vi "fgv_Sys Config.vi"(7 "Standalone viewer initialisation?":bool, 8 "error in (no error)":errorcluster, 10 "Function":T11, 11 "System Config in":T1={"XY Stage"={"COM port"="", "XY stage available"=FALSE, "Baudrate"=0, "Type"=""}, "DAQ FPGA"={"Target"="RIO0", "input card type"=enum."AC Card", "Ref"=refnum, "Clock Freq (MHz) "=200.0, "Samples Wait after Trigger"=5080, "AOD fill"=4900, "StartupDelay"=0, "Slip Cycle (clock cycles)"=600000, "Add Cycle"=TRUE}, "Control system"={"Ctrl FPGA available"=FALSE, "Control system.FPGA Type"="", "Control system.Network adapter name"="", "Control system.MAC address"="", "Control system.Ethernet Port"=3, "Ethernet opened"=FALSE, "Ctrl FPGA Clock (MHz)"=240.0, "AOD 1 Amplitude"=0, "AOD 2 Amplitude"=0, "AOD 3 Amplitude"=0, "AOD 4 Amplitude"=0, "AOD 5 Amplitude"=0, "AOD 6 Amplitude"=0, "Data Time Interval (ns)"=0.0, "T0 (ns)"=0.0, "Ta (ns)"=0.0, "Ethernet Port"=3}, "Encoder"={"IP address"="224.0.1.103", "Port"=7000, "Encoder available"=FALSE, "Wheel radius (cm)"=16.0, "Encoder Trigger"=""}, "DAQmx Chan"={"Pockels AO"="", "Hard shutter AO"="", "PMT AOs"="", "Galvo AOs"="", "Power meter AI"=""}, "Computer MAC address"="", "Cam VidRec"={"DO flag-Video record"="", "DO flag-Trial start"="", "VidRec available"=FALSE}, "Externalise Triggers"=FALSE, "MC Supported"=FALSE, "Laser wavelength (nm)"=920.0} {"Laser wavelength (nm)" min=800.0 max=1080.0 step=1.0; "Encoder"."Wheel radius (cm)" format="%#_13g"; "Control system"."Control system.Ethernet Port" min=0 max=2048 step=1; "Control system"."Ctrl FPGA Clock (MHz)" min=80.0 max=500.0 step=1.0; "Control system"."Data Time Interval (ns)" min=0.0 max=2048.0 step=1.0; "Control system"."Ta (ns)" min=0.0 max=2048.0 step=1.0; "Control system"."T0 (ns)" min=0.0 max=2048.0 step=1.0; "Control system"."AOD 6 Amplitude" min=0 max=2048 step=1; "Control system"."AOD 5 Amplitude" min=0 max=2048 step=1; "Control system"."AOD 4 Amplitude" min=0 max=2048 step=1; "Control system"."AOD 3 Amplitude" min=0 max=2048 step=1; "Control system"."AOD 2 Amplitude" min=0 max=2048 step=1; "Control system"."AOD 1 Amplitude" min=0 max=2048 step=1}) -> (0 "error out":errorcluster, 3 "System Config out":T1={"XY Stage"={"COM port"="", "XY stage available"=FALSE, "Baudrate"=0, "Type"=""}, "DAQ FPGA"={"Target"="RIO0", "input card type"=enum."AC Card", "Ref"=refnum, "Clock Freq (MHz) "=200.0, "Samples Wait after Trigger"=5080, "AOD fill"=4900, "StartupDelay"=0, "Slip Cycle (clock cycles)"=600000, "Add Cycle"=TRUE}, "Control system"={"Ctrl FPGA available"=FALSE, "Control system.FPGA Type"="", "Control system.Network adapter name"="", "Control system.MAC address"="", "Control system.Ethernet Port"=3, "Ethernet opened"=FALSE, "Ctrl FPGA Clock (MHz)"=240.0, "AOD 1 Amplitude"=0, "AOD 2 Amplitude"=0, "AOD 3 Amplitude"=0, "AOD 4 Amplitude"=0, "AOD 5 Amplitude"=0, "AOD 6 Amplitude"=0, "Data Time Interval (ns)"=0.0, "T0 (ns)"=0.0, "Ta (ns)"=0.0, "Ethernet Port"=3}, "Encoder"={"IP address"="224.0.1.103", "Port"=7000, "Encoder available"=FALSE, "Wheel radius (cm)"=16.0, "Encoder Trigger"=""}, "DAQmx Chan"={"Pockels AO"="", "Hard shutter AO"="", "PMT AOs"="", "Galvo AOs"="", "Power meter AI"=""}, "Computer MAC address"="", "Cam VidRec"={"DO flag-Video record"="", "DO flag-Trial start"="", "VidRec available"=FALSE}, "Externalise Triggers"=FALSE, "MC Supported"=FALSE, "Laser wavelength (nm)"=920.0} {"Laser wavelength (nm)" min=800.0 max=1080.0 step=1.0; "Encoder"."Wheel radius (cm)" format="%#_13g"; "Control system"."Control system.Ethernet Port" min=0 max=2048 step=1; "Control system"."Ctrl FPGA Clock (MHz)" min=80.0 max=500.0 step=1.0; "Control system"."Data Time Interval (ns)" min=0.0 max=2048.0 step=1.0; "Control system"."Ta (ns)" min=0.0 max=2048.0 step=1.0; "Control system"."T0 (ns)" min=0.0 max=2048.0 step=1.0; "Control system"."AOD 6 Amplitude" min=0 max=2048 step=1; "Control system"."AOD 5 Amplitude" min=0 max=2048 step=1; "Control system"."AOD 4 Amplitude" min=0 max=2048 step=1; "Control system"."AOD 3 Amplitude" min=0 max=2048 step=1; "Control system"."AOD 2 Amplitude" min=0 max=2048 step=1; "Control system"."AOD 1 Amplitude" min=0 max=2048 step=1})   [LabVIEW 2017]
uses:
  Typedefs/Save-Load enum.ctl
  General Globals.vi
  <vilib>/userdefined/High Color/nirio_resource_hc.ctl
  Typedefs/DAQ FPGA config cluster.ctl
  Typedefs/DAQmx physical channels cluster.ctl
  Typedefs/CTRL system config cluster.ctl
  Typedefs/Sys Configuration.ctl
  Typedefs/XY Stage config cluster.ctl
  Typedefs/HW config states enum.ctl
  RIG-SPECIFIC FILES/FPGA Refs/FPGA Ref.ctl
  Typedefs/FPGA input type AC-DC.ctl
  Typedefs/Encoder config cluster.ctl
  Typedefs/Cam VidRec HW config setup cluster.ctl
panel:
  # "FUNCTIONAL GLOBAL"
  # "<--- The \"PMT AOs\" DAQmx string will always contain\n                       2 channels is this format: PXI1Slot4/ao2:3"
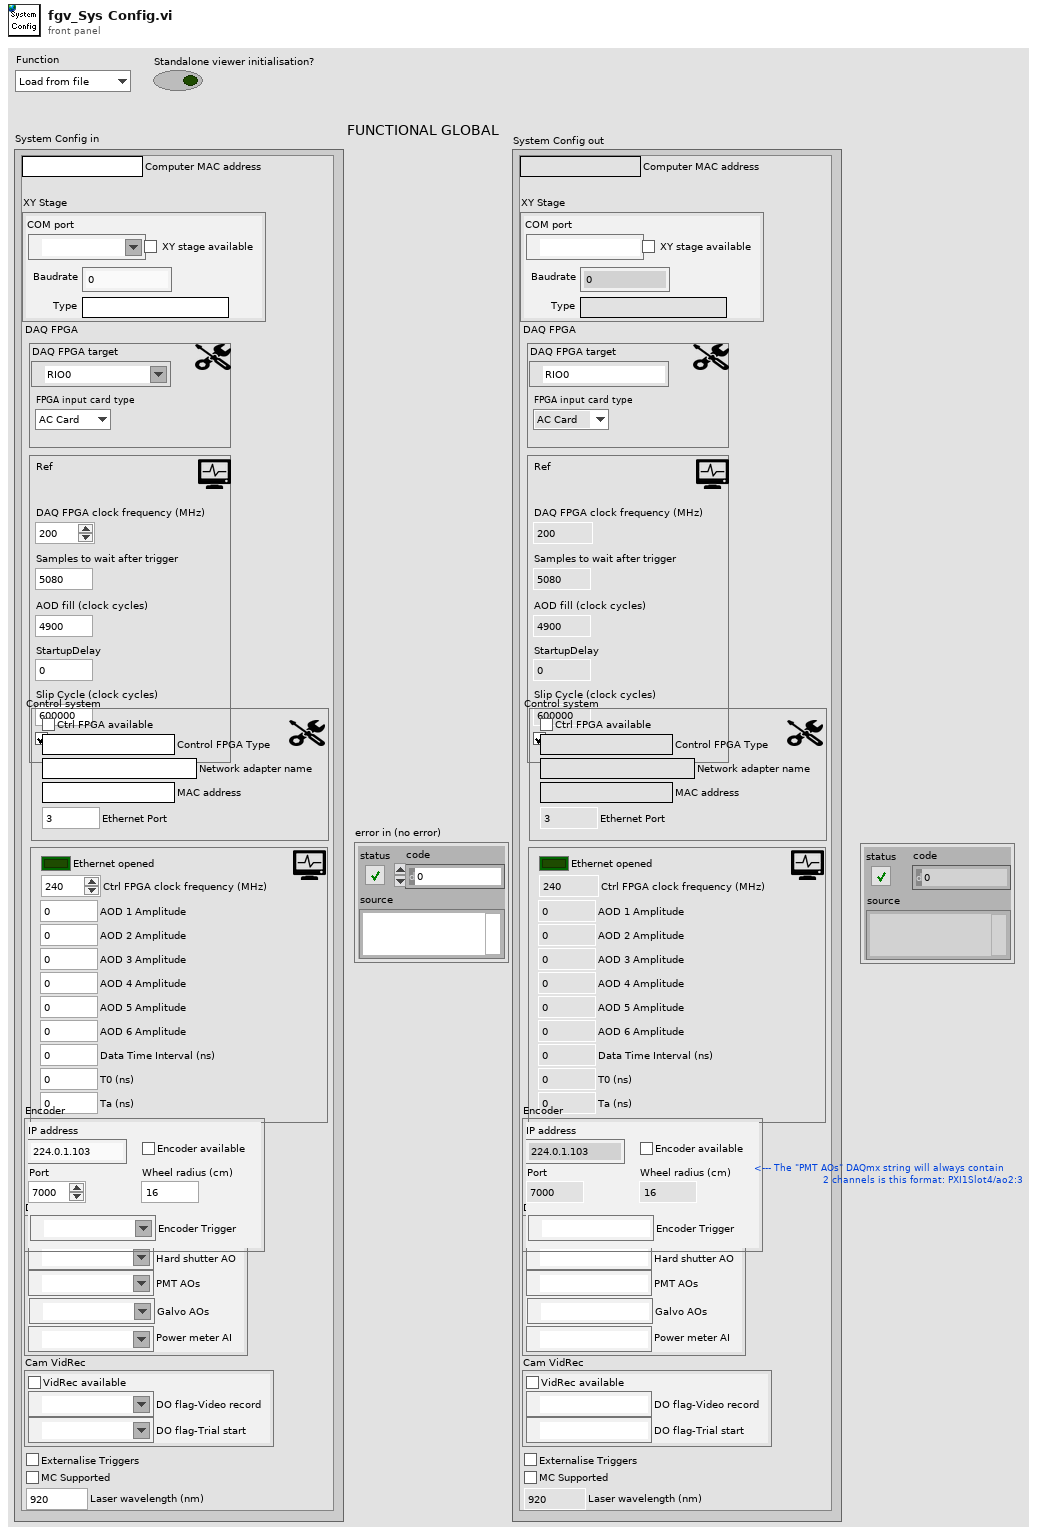
[diagram p1: front panel]
types:
  T1 = typedef "Sys Configuration.ctl" = cluster{"XY Stage":T2, "DAQ FPGA":T3, "Control system":T7, "Encoder":T8, "DAQmx Chan":T9, "Computer MAC address":string, "Cam VidRec":T10, "Externalise Triggers":bool, "MC Supported":bool, "Laser wavelength (nm)":dbl}
  T2 = typedef "XY Stage config cluster.ctl" = cluster{"COM port":refnum<visa-resource-name>, "XY stage available":bool, "Baudrate":i32, "Type":string}
  T3 = typedef "DAQ FPGA config cluster.ctl" = cluster{"Target":T4, "input card type":T5, "Ref":T6, "Clock Freq (MHz) ":dbl, "Samples Wait after Trigger":u16, "AOD fill":u16, "StartupDelay":i32, "Slip Cycle (clock cycles)":u32, "Add Cycle":bool}
  T4 = typedef "nirio_resource_hc.ctl" = tag
  T5 = typedef "FPGA input type AC-DC.ctl" = enum16{"AC Card", "DC Card"}
  T6 = typedef "FPGA Ref.ctl" = refnum<k20>
  T7 = typedef "CTRL system config cluster.ctl" = cluster{"Ctrl FPGA available":bool, "Control system.FPGA Type":string, "Control system.Network adapter name":string, "Control system.MAC address":string, "Control system.Ethernet Port":i16, "Ethernet opened":bool, "Ctrl FPGA Clock (MHz)":dbl, "AOD 1 Amplitude":i16, "AOD 2 Amplitude":i16, "AOD 3 Amplitude":i16, "AOD 4 Amplitude":i16, "AOD 5 Amplitude":i16, "AOD 6 Amplitude":i16, "Data Time Interval (ns)":dbl, "T0 (ns)":dbl, "Ta (ns)":dbl, "Ethernet Port":u32}
  T8 = typedef "Encoder config cluster.ctl" = cluster{"IP address":string, "Port":u16, "Encoder available":bool, "Wheel radius (cm)":dbl, "Encoder Trigger":tag}
  T9 = typedef "DAQmx physical channels cluster.ctl" = cluster{"Pockels AO":tag, "Hard shutter AO":tag, "PMT AOs":tag, "Galvo AOs":tag, "Power meter AI":tag}
  T10 = typedef "Cam VidRec HW config setup cluster.ctl" = cluster{"DO flag-Video record":tag, "DO flag-Trial start":tag, "VidRec available":bool}
  T11 = typedef "HW config states enum.ctl" = enum16{"Load from file", "Save to file", "Write all", "Read all", "Write XY stage settings", "Write DAQ FPGA settings", "Write Control FPGA settings", "Write Phys Channels", "Clear", "Compare from file"}
  T12 = typedef "Save-Load enum.ctl" = enum16{"Save to file", "Load from file", "Compare from file"}
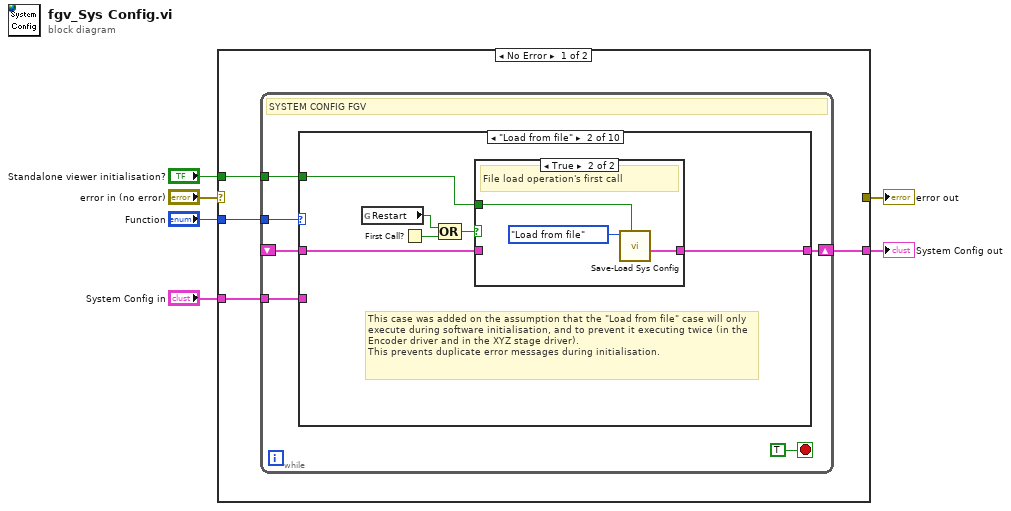
[diagram p0: block diagram]
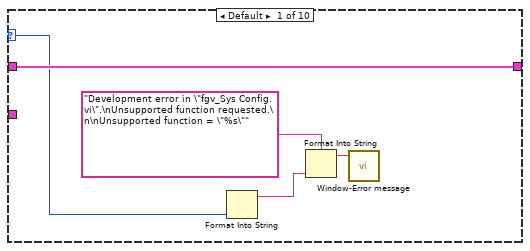
[diagram p2: hidden frame]
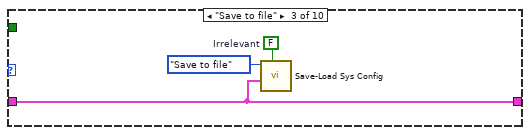
[diagram p4: hidden frame]
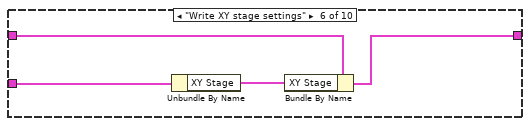
[diagram p7: hidden frame]
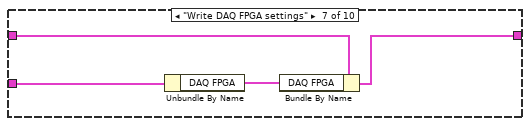
[diagram p8: hidden frame]
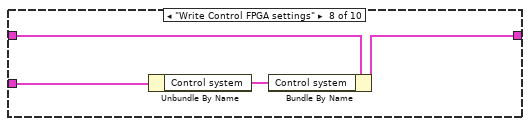
[diagram p9: hidden frame]
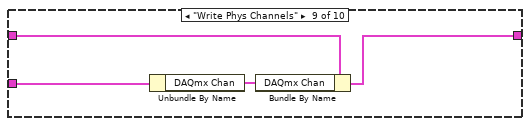
[diagram p10: hidden frame]
diagram:
  n1 = case shown="No Error" "error in (no error)" {
    selector: "error in (no error)" -> [_ w53]
    tunnel: [_ w53] -> w5
    tunnel: "Function" -> [w10 _]
    tunnel: "System Config in" -> [w9 _]
    tunnel: [w8 _] -> w2
    tunnel: "Standalone viewer initialisation?" -> [w7 _]
    frame No Error {
      n2 = while {
        tunnel: w10 -> [w16]
        shift-right: [w14] -> w8
        shift-left: _ -> [w12]
        tunnel: w9 -> [w13]
        tunnel: w7 -> [w11]
        stop <- TRUE stop-if-true
        # "SYSTEM CONFIG FGV"
        n3 = case shown="\"Load from file\"" w16 {
          selector: w16 -> [w17 _ _ _ _ _ _ _ _ _]
          tunnel: [w18 w27 w34 w35 w36 w37 w41 w45 w49 _] -> w14
          tunnel: w13 -> [_ _ _ w35 _ w40 w44 w48 w52 _]
          tunnel: w12 -> [w18 w26 w34 _ w36 w39 w43 w47 w51 _]
          tunnel: w11 -> [_ w22 _ _ _ _ _ _ _ _]
          frame Default {
            n4 = Format Into String(w17) -> (resulting string=w20:string)  [unwired: 3 in, 1 out]
            n5 = Format Into String(format string="Development error in \"fgv_Sys Config.vi\".\nUnsupported function requested.\n\nUnsupported function = \"%s\"" ("Message"), w20) -> (resulting string=w19:string)  [unwired: 2 in, 1 out]
            n6 = call "Window-Error message.vi"("Message"=w19) -> ()  [unwired: 10 in, 1 out]
          }
          frame "Load from file" {
            # "This case was added on the assumption that the \"Load from file\" case will only execute during software initialisation, and to prevent it executing twice (in the Encoder driver and in the XYZ stage driver).\nThis prevents duplicate error messages during initialisation."
            n7 = global read "General Globals.vi" "Restart"() -> (w23:bool)
            n8 = First Call?() -> (First Call?: T/F=w25:bool)
            n9 = Compound Arithmetic op=OR(w23, w25) -> (w24:bool)
            n10 = case shown="True" w24 {
              tunnel: [w28 w31] -> w27
              tunnel: w26 -> [w28 _]
              tunnel: w22 -> [_ w29]
              frame False {
                # "Already loaded"
              }
              frame True {
                # "File load operation's first call"
                n11 = call "Save-Load Sys Config.vi"("Standalone viewer?"=w29, "Function"=Save-Load_enum."Load from file") -> ("Loaded System config"=w31:T1)  [unwired: 8 in, 1 out]
              }
            }
          }
          frame "Save to file" {
            w32 = FALSE  # Irrelevant
            n12 = call "Save-Load Sys Config.vi"("Standalone viewer?"=w32, "System config to save"=w34, "Function"=Save-Load_enum."Save to file") -> ()  [unwired: 7 in, 2 out]
          }
          frame "Write all" {
          }
          frame "Read all" {
          }
          frame "Write XY stage settings" {
            n13 = Unbundle By Name(w40) -> ("XY Stage"=w38:T2)
            n14 = Bundle By Name(cluster=w39, "XY Stage"=w38) -> (w37:T1)
          }
          frame "Write DAQ FPGA settings" {
            n15 = Unbundle By Name(w44) -> ("DAQ FPGA"=w42:T3)
            n16 = Bundle By Name(cluster=w43, "DAQ FPGA"=w42) -> (w41:T1)
          }
          frame "Write Control FPGA settings" {
            n17 = Unbundle By Name(w48) -> ("Control system"=w46:T7)
            n18 = Bundle By Name(cluster=w47, "Control system"=w46) -> (w45:T1)
          }
          frame "Write Phys Channels" {
            n19 = Unbundle By Name(w52) -> ("DAQmx Chan"=w50:T9)
            n20 = Bundle By Name(cluster=w51, "DAQmx Chan"=w50) -> (w49:T1)
          }
          frame "Clear" {
          }
        }
      }
    }
    frame Error {
    }
  }
  "error out" <- w5
  "System Config out" <- w2
